vi "Config CanCoder Set.vi"(5 "Max # Of Tries":i32=5, 6 "Send Cmd Timout(ms)":u32=300, 7 "CAN":T1, 8 "Error":errorcluster, 9 "Can Coder Data":T2={"ID"=0, "Zero Offset"=0.0, "CW(t) CCW(f)"=TRUE}, 11 "CANcoder Ref":T3) -> (0 "Error Out":errorcluster, 3 "CANcoder Ref Out":T3)   [LabVIEW 2020, in "Wrist_ACT.lvlib"]
uses:
  <vilib>/Rock Robotics/WPI/ThirdParty/Phoenix-LabVIEW/CANCoder/Controls/CTRE_Phoenix_CANcoder_DeviceRef.ctl
  Shared Code/TypeDefs/Cluster_Config_Cancoder Data.ctl
  Shared Code/TypeDefs/Cluser_CAN Data.ctl
  <vilib>/Rock Robotics/WPI/ThirdParty/Phoenix-LabVIEW/CANCoder/Controls/CTRE_Phoenix_CANcoder_AbsoluteSensorRange.ctl
  <vilib>/Rock Robotics/WPI/ThirdParty/Phoenix-LabVIEW/CANCoder/Controls/CTRE_Phoenix_CANcoder_SensorInitializationStrategy.ctl
  <vilib>/Rock Robotics/WPI/ThirdParty/Phoenix-LabVIEW/CANCoder/Set/CTRE_Phoenix_CANcoder_SetPositionToAbsolute.vi
  Wrist_ACT.lvlib
  <vilib>/Utility/Data Type/NI_Data Type.lvlib
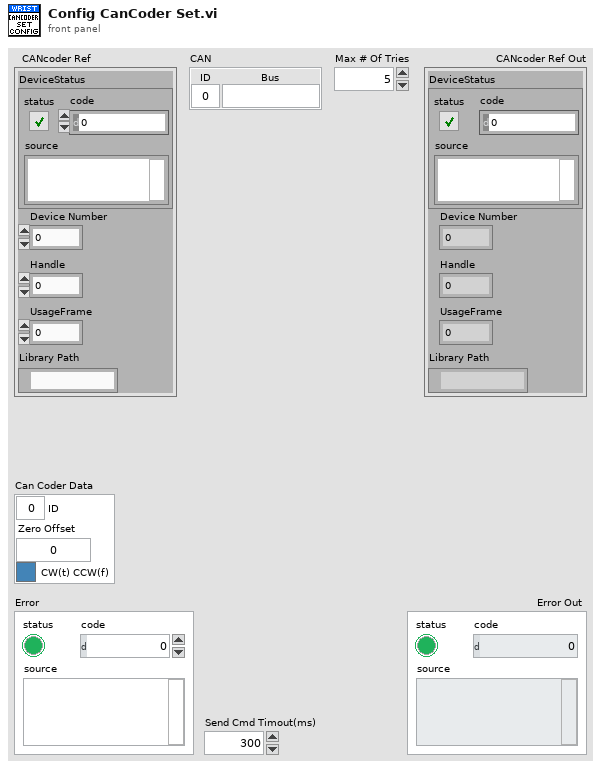
[diagram p1: front panel]
types:
  T1 = typedef "Cluser_CAN Data.ctl" = cluster{"ID":u8, "Bus":string}
  T2 = typedef "Cluster_Config_Cancoder Data.ctl" = cluster{"ID":u8, "Zero Offset":dbl, "CW(t) CCW(f)":bool}
  T3 = typedef "CTRE_Phoenix_CANcoder_DeviceRef.ctl" = cluster{"DeviceStatus":errorcluster, "Device Number":u8, "Handle":u64, "UsageFrame":u32, "Library Path":path}
  T4 = typedef "CTRE_Phoenix_CANcoder_SensorInitializationStrategy.ctl" = enum16{"Boot To Zero", "Boot To Absolute Position"}
  T5 = typedef "CTRE_Phoenix_CANcoder_AbsoluteSensorRange.ctl" = enum16{"Unsigned [0 to 360)", "Signed [-180 to +180)"}
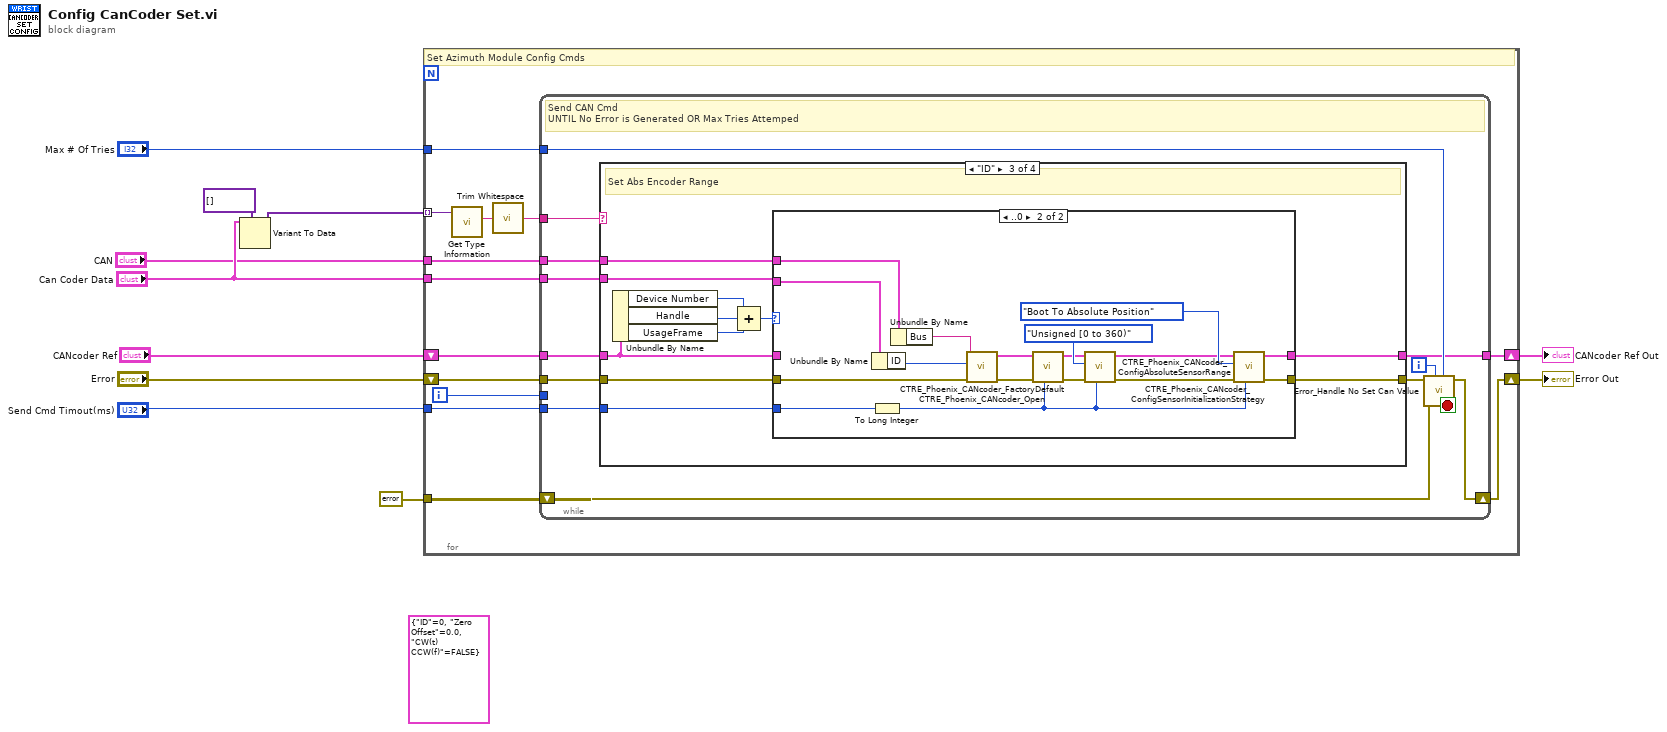
[diagram p0: block diagram]
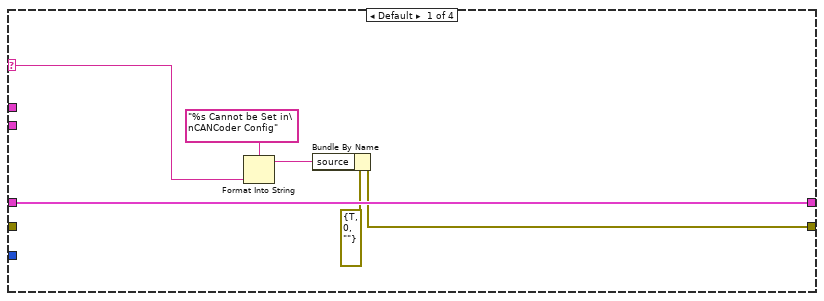
[diagram p2: hidden frame]
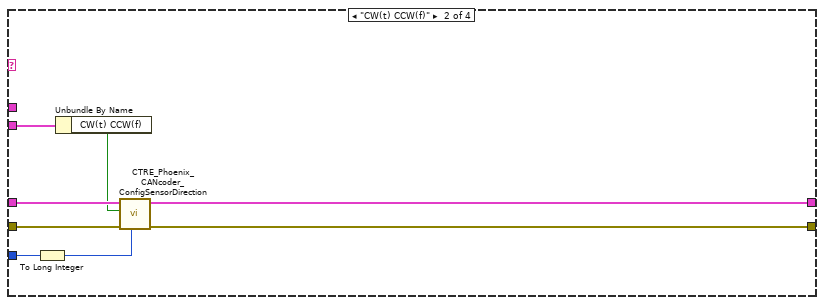
[diagram p3: hidden frame]
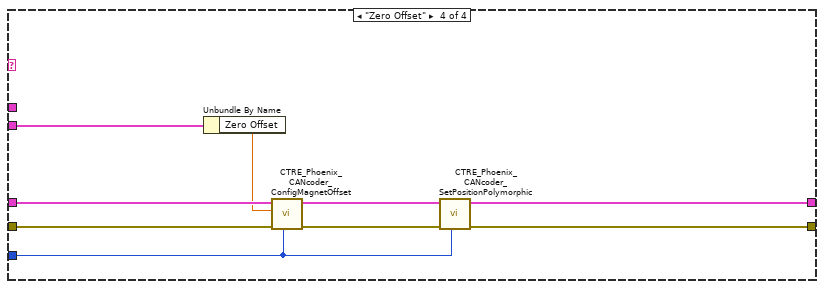
[diagram p5: hidden frame]
diagram:
  (unwired) T2 {"ID"=0, "Zero Offset"=0.0, "CW(t) CCW(f)"=FALSE} ("Can Coder Data")
  n1 = Variant To Data(type=variant[] [], Variant="Can Coder Data") -> (data=w2:variant[])  [unwired: 1 in, 1 out]
  n2 = for {
    tunnel: errorcluster {"status"=FALSE, "code"=0, "source"=""} ("Error Out") -> [w22]
    shift-right: [w23] -> w11
    shift-left: "Error" -> [w20]
    shift-right: [w24] -> w9
    shift-left: "CANcoder Ref" -> [w21]
    tunnel: "Max # Of Tries" -> [w18]
    tunnel: w2 -> [w16] mode=indexing
    tunnel: "Send Cmd Timout(ms)" -> [w14]
    tunnel: "Can Coder Data" -> [w13]
    tunnel: "CAN" -> [w12]
    i -> [w19]
    # "Set Azimuth Module Config Cmds"
    n3 = call <vilib>:"Get Type Information.vi"("variant"=w16) -> ("name"=w17:string)  [unwired: 6 in, 4 out]
    n4 = call <vilib>:"Trim Whitespace.vi"("string"=w17) -> ("trimmed string"=w15:string)  [unwired: 1 in]
    n5 = while {
      tunnel: [w28] -> w24
      tunnel: w14 -> [w34]
      shift-right: [w36] -> w23
      shift-left: w22 -> [w33]
      tunnel: w20 -> [w31]
      tunnel: w21 -> [w30]
      tunnel: w19 -> [_]
      tunnel: w18 -> [w29]
      tunnel: w15 -> [w27]
      tunnel: w13 -> [w26]
      tunnel: w12 -> [w25]
      i -> [w32]
      stop <- w35 stop-if-true
      # "Send CAN Cmd\nUNTIL No Error is Generated OR Max Tries Attemped"
      n6 = case shown="\"ID\"" w27 {
        selector: w27 -> [w41 _ _ _]
        tunnel: [w38 w49 w61 w83] -> w37
        tunnel: w34 -> [_ w47 w60 w85]
        tunnel: w31 -> [_ w48 w62 w84]
        tunnel: w30 -> [w40 w51 w53 w89]
        tunnel: [w40 w50 w59 w87] -> w28
        tunnel: w26 -> [_ w44 w58 w82]
        tunnel: w25 -> [_ _ w52 _]
        frame Default {
          n7 = Format Into String(format string="%s Cannot be Set in\nCANCoder Config", w41) -> (resulting string=w42:string)  [unwired: 2 in, 1 out]
          n8 = Bundle By Name(cluster=errorcluster {"status"=TRUE, "code"=0, "source"=""} ("error out"), "source"=w42) -> (w38:errorcluster)
        }
        frame "CW(t) CCW(f)" {
          n9 = To Long Integer(number=w47) -> (32bit integer=w45:i32)
          n10 = Unbundle By Name(w44) -> ("CW(t) CCW(f)"=w46:bool)
          n11 = call <vilib>:"CTRE_Phoenix_CANcoder_ConfigSensorDirection.vi"("timeoutMs"=w45, "error in"=w48, "Sensor Direction"=w46, "CTRE_CANcoder_DeviceRef"=w51) -> ("error out"=w49:errorcluster, "CTRE_CANcoder_DeviceRef"=w50:T3)  [unwired: 6 in]
        }
        frame "ID" {
          # "Set Abs Encoder Range"
          n12 = Unbundle By Name(w53) -> ("Device Number"=w56:u8, "Handle"=w57:u64, "UsageFrame"=w55:u32)
          n13 = Compound Arithmetic op=ADD(w56, w57, w55) -> (w54:u64)
          n14 = case shown="..0" w54 {
            tunnel: w62 -> [w64 w80]
            tunnel: [w64 w72] -> w61
            tunnel: w60 -> [_ w71]
            tunnel: [w63 w69] -> w59
            tunnel: w58 -> [_ w67]
            tunnel: w53 -> [w63 _]
            tunnel: w52 -> [_ w66]
            frame 1.. {
            }
            frame ..0 {
              n15 = Unbundle By Name(w67) -> ("ID"=w79:u8)
              n16 = To Long Integer(number=w71) -> (32bit integer=w68:i32)
              n17 = Unbundle By Name(w66) -> ("Bus"=w65:string)
              n18 = call <vilib>:"CTRE_Phoenix_CANcoder_Open.vi"("error in"=w80, "Device Number"=w79, "CAN Bus"=w65) -> ("error out"=w76:errorcluster, "CTRE_CANcoder_DeviceRef"=w78:T3)  [unwired: 7 in]
              n19 = call <vilib>:"CTRE_Phoenix_CANcoder_FactoryDefault.vi"("timeoutMs"=w68, "error in"=w76, "CTRE_CANcoder_DeviceRef"=w78) -> ("error out"=w75:errorcluster, "CTRE_CANcoder_DeviceRef"=w77:T3)  [unwired: 7 in]
              n20 = call <vilib>:"CTRE_Phoenix_CANcoder_ConfigAbsoluteSensorRange.vi"("timeoutMs"=w68, "error in"=w75, "Absolute Sensor Range"=CTRE_Phoenix_CANcoder_AbsoluteSensorRange."Unsigned [0 to 360)", "CTRE_CANcoder_DeviceRef"=w77) -> ("error out"=w73:errorcluster, "CTRE_CANcoder_DeviceRef"=w70:T3)  [unwired: 6 in]
              n21 = call <vilib>:"CTRE_Phoenix_CANcoder_ConfigSensorInitializationStrategy.vi"("timeoutMs"=w68, "error in"=w73, "Sensor Initialization Strategy"=CTRE_Phoenix_CANcoder_SensorInitializationStrategy."Boot To Absolute Position", "CTRE_CANcoder_DeviceRef"=w70) -> ("error out"=w72:errorcluster, "CTRE_CANcoder_DeviceRef"=w69:T3)  [unwired: 6 in]
            }
          }
        }
        frame "Zero Offset" {
          n22 = Unbundle By Name(w82) -> ("Zero Offset"=w88:dbl)
          n23 = call <vilib>:"CTRE_Phoenix_CANcoder_ConfigMagnetOffset.vi"("timeoutMs"=w85, "error in"=w84, "Magnet Offset (Degrees)"=w88, "CTRE_CANcoder_DeviceRef"=w89) -> ("error out"=w86:errorcluster, "CTRE_CANcoder_DeviceRef"=w90:T3)  [unwired: 6 in]
          n24 = call-poly <vilib>:"CTRE_Phoenix_CANcoder_SetPositionPolymorphic.vi"("timeoutMs"=w85, "error in (no error)"=w86, "CTRE_CANcoder_DeviceRef"=w90) -> ("error out"=w83:errorcluster, "CTRE_CANcoder_DeviceRef"=w87:T3)  [unwired: 7 in]
        }
      }
      n25 = call "Error_Handle No Set Can Value.vi"("Max # Of Tries"=w29, "Loop Itteration"=w32, "Previous Error"=w33, "Error"=w37) -> ("Stop Out"=w35:bool, "Error Out"=w36:errorcluster)  [unwired: 6 in]
    }
  }
  "Error Out" <- w11
  "CANcoder Ref Out" <- w9
